vi "YokogawaGS200ReadAlex.vi"(2 "Point #":i32, 3 "Parameters":dbl[](array[numeric]) format="%.3e", 4 "Instrument Address":refnum<visa-resource-name>) -> (0 "Stop":bool, 1 "Measurement":dbl[](array[numeric]) format="%.6e")   [LabVIEW 2024]
doc: "This VI reads a single reading from a Keithley 2001 multimeter. The stop boolean is always false. If no reading is obtained a single zero is returned.\nScott Hannahs, NHMFL-FSU, Nov 1993"
panel:
  # "The zero parameter tells it\nto read the source value if =0\nto read the measur. result if =1"
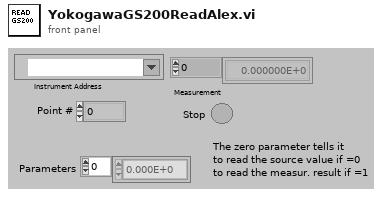
[diagram p1: front panel]
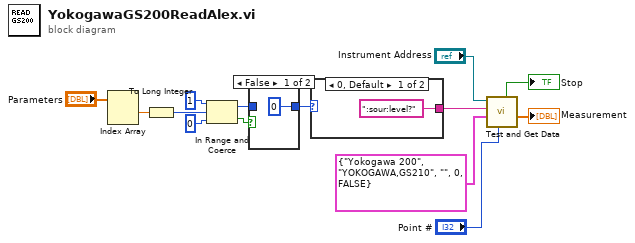
[diagram p0: block diagram]
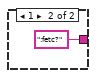
[diagram p3: hidden frame]
diagram:
  n1 = Index Array(array="Parameters") -> (element #1=w6:dbl)  [unwired: 2 in, 1 out]
  n2 = To Long Integer(number=w6) -> (32bit integer=w5:i32)
  n3 = In Range and Coerce(upper limit=1, x=w5, lower limit=0) -> (coerced(x)=w3:i32, In Range?=w4:bool)
  n4 = case shown="False" w4 {
    tunnel: w3 -> [_ w16]
    tunnel: [0 w16] -> w2
    frame False {
    }
    frame True {
    }
  }
  n5 = case shown="0, Default" w2 {
    tunnel: [":sour:level?" ":fetc?"] -> w1
    frame 0, Default {
    }
    frame 1 {
    }
  }
  n6 = call "Test and Get Data.vi"("Point #"="Point #", "Instrument Info"=cluster{string, string, string, u32, bool} {"Yokogawa 200", "YOKOGAWA,GS210", "", 0, FALSE}, "Command String"=w1, "VISA Sesson"="Instrument Address") -> ("Measurement"=→"Measurement":dbl[], "Stop"=→"Stop":bool)  [unwired: 2 in, 3 out]
